vi "提取日志报警参数入列队 (子VI).vi"(10 "枚举":T1(ring), 11 "queue in":refnum<queue>) -> ()   [LabVIEW 2016]
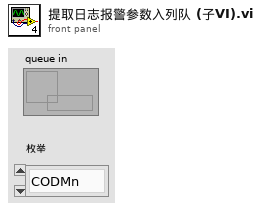
[diagram p1: front panel]
types:
  T1 = enum16{"CODMn", "CODCr", "氨氮", "总磷", "总氮", "数采仪"}
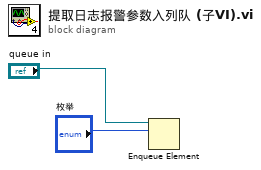
[diagram p0: block diagram]
diagram:
  n1 = Enqueue Element(queue="queue in", element="枚举") -> ()  [unwired: 2 in, 3 out]
